vi "71 MP_Reading a voltage.vi"() -> ()   [LabVIEW 2019]
uses:
  <vilib>/Instr/_visa.llb/VISA Configure Serial Port (Instr).vi
  _Subs/OpenDiagram/Open_XControl.xctl
panel:
  out "Connected":bool=TRUE
  in  "stop":bool
  in  "MicroPython code":string="'''\nhttps://docs.micropython.org/en/latest/\n     \nconnections: \nGround (B) - GND \nSignal -  pin X1\n'''\n\nimport pyb,utime\n\nusb = pyb.USB_VCP()\nadc = pyb.ADC(pyb.Pin.board.X2)    \n\nwhile True:\n     value = adc.read()\n     string = '%d \\n' % (value)\n     usb.send(string)\n     utime.sleep_ms(100)"
  in  "MicroPython Port":refnum<visa-resource-name>="ASRL96::INSTR"
  out "Gauge":i32(knob) scale=0.0..1000.0
  in  "OpenDiag":refnum<vi>(xcontrol)
  # "01 MicroPython Reading a Voltage\nThis code takes will read a voltage from your MicroPython Device\n\nInstructions:\n1. Download the MicroPython Code into your device by saving it as main.py on your device\n2. restart your device\n3. Select the device port \n4. Hit Run - and watch the gauge change value with the sensor"
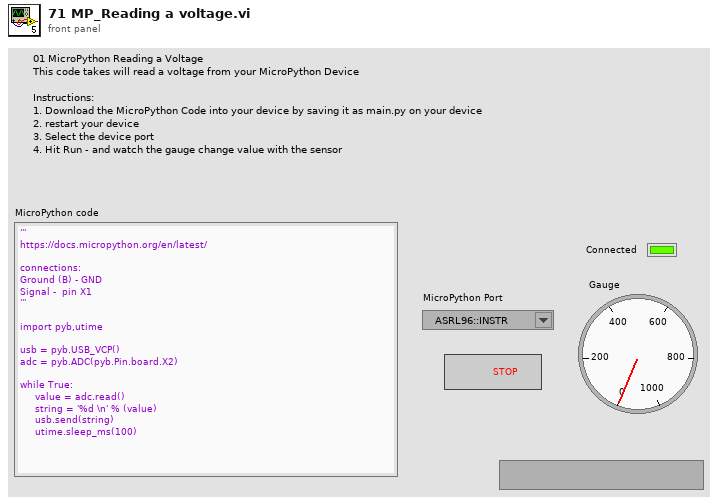
[diagram p1: front panel]
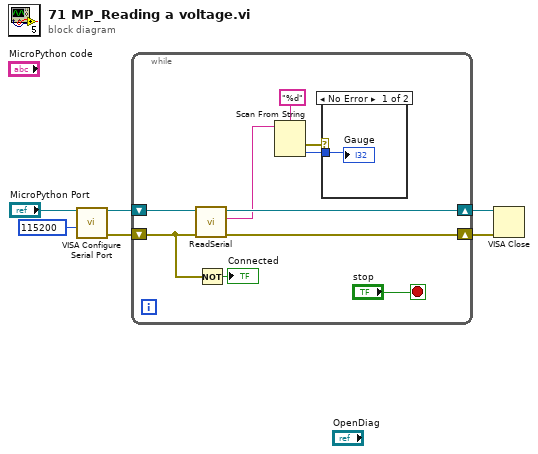
[diagram p0: block diagram]
diagram:
  n1 = call-poly "VISA Configure Serial Port"("VISA resource name"="MicroPython Port", "baud rate (9600)"=u32 115200) -> ("VISA resource name out"=w5:refnum<visa-resource-name>, "error out"=w4:errorcluster)  [unwired: 12 in]
  n2 = while {
    shift-right: [w9] -> w2
    shift-left: w5 -> [w10]
    shift-right: [w8] -> w3
    shift-left: w4 -> [w11]
    stop <- "stop" stop-if-true
    n3 = call "ReadSerial.vi"("error in (no error)"=w11, "VISA Refnum in"=w10) -> ("error out"=w8:errorcluster, "String"=w7:string, "VISA Refnum out"=w9:refnum<visa-resource-name>)  [unwired: 7 in]
    n4 = Not(x=w11) -> (.not. x?=→"Connected":bool)
    n5 = Scan From String(format string="%d", input string=w7) -> (error out=w13:errorcluster, output 1=w12:i32)  [unwired: 3 in, 2 out]
    n6 = case shown="No Error" w13 {
      tunnel: w12 -> [w17 _]
      frame No Error {
        "Gauge" <- w17
      }
      frame Error {
      }
    }
  }
  n7 = VISA Close(VISA resource name=w2, error in (no error)=w3) -> ()  [unwired: 1 out]
